vi "Simple_PI.vi"(9 "Current":dbl, 10 "Desired":dbl, 11 "input cluster":T1) -> (3 "Y":dbl)   [LabVIEW 2019]
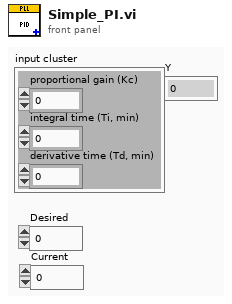
[diagram p1: front panel]
types:
  T1 = cluster{"proportional gain (Kc)":dbl, "integral time (Ti, min)":dbl, "derivative time (Td, min)":dbl}
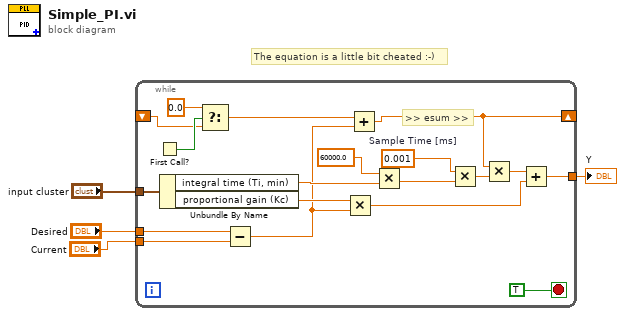
[diagram p0: block diagram]
diagram:
  # "The equation is a little bit cheated :-)"
  n1 = while {
    tunnel: "input cluster" -> [w15]
    tunnel: "Desired" -> [w14]
    tunnel: "Current" -> [w13]
    shift-right: [w5] -> _
    shift-left: _ -> [w10]
    tunnel: [w6] -> w1
    stop <- TRUE stop-if-true
    w22 = 0.001  # Sample Time [ms]
    # ">> esum >>"
    n2 = First Call?() -> (First Call?: T/F=w11:bool)
    n3 = Unbundle By Name(w15) -> ("integral time (Ti, min)"=w18:dbl, "proportional gain (Kc)"=w23:dbl)
    n4 = Select(t=0.0, s=w11, f=w10) -> (s? t:f=w8:dbl)
    n5 = Subtract(x=w14, y=w13) -> (x-y=w7:dbl)
    n6 = Multiply(x=w23, y=w7) -> (x*y=w19:dbl)
    n7 = Add(x=w8, y=w7) -> (x+y=w5:dbl)
    n8 = Multiply(x=60000.0, y=w18) -> (x*y=w16:dbl)
    n9 = Multiply(x=w22, y=w16) -> (x*y=w21:dbl)
    n10 = Multiply(x=w5, y=w21) -> (x*y=w20:dbl)
    n11 = Add(x=w20, y=w19) -> (x+y=w6:dbl)
  }
  "Y" <- w1
